vi "hw4-2 topVI.vi"() -> ()   [LabVIEW 2014]
uses:
  <vilib>/regexp/Match Regular Expression.xnode
panel:
  in  "file path (use dialog)":path
  out "output":string[][](array[string])
  in  "Firewall log raw data":string="Apr 26 21:31:34 filterlog: 129,16777216,,1425041642,hn0,match,pass,in,4,0x0,,128,16110,0,none,17,udp,36,10.2.10.175,255.255.255.255,60221,3956,16\nApr 26 21:31:34 filterlog: 129,16777216,,1425041642,hn0,match,pass,in,4,0x0,,128,4117,0,none,17,udp,78,10.2.10.1,208.93.4.206,137,137,58\nApr 26 21:31:32 filterlog: 130,16777216,,1425041643,hn0,match,pass,in,4,0x0,,128,18168,0,DF,17,udp,351,10.2.10.10,10.2.23.123,53,59118,331\nApr 26 21:31:32 filterlog: 129,16777216,,1425041642,hn0,match,pass,in,4,0x0,,128,10627,0,none,17,udp,82,10.2.10.10,140.112.2.2,59087,53,62\nApr 26 21:31:32 filterlog: 129,16777216,,1425041642,hn0,match,pass,in,4,0x0,,128,10626,0,none,17,udp,98,10.2.10.10,140.112.2.2,60847,53,78\nApr 26 21:38:10 filterlog: 105,16777216,,1425041627,hn1,match,block,in,4,0x2,0,109,9812,0,DF,6,tcp,48,207.46.13.171,10.2.10.15,25309,80,0,SEC,27892632,,8192,,mss;nop;nop;sackOK\nApr 26 21:38:08 filterlog: 129,16777216,,1425041642,hn0,match,pass,in,4,0x0,,128,23124,0,DF,6,tcp,52,10.2.10.172,207.46.153.155,60590,443,0,S,2141064781,,8192,,mss;nop;wscale;nop;nop;sackOK\nApr 26 21:38:08 filterlog: 130,16777216,,1425041643,hn0,match,block,in,4,0x2,0,128,8596,0,DF,6,tcp,48,10.2.10.2,10.2.102.10,41875,88,0,SEC,3256166066,,8192,,mss;nop;nop;sackOK\nApr 26 21:38:07 filterlog: 130,16777216,,1425041643,hn0,match,pass,in,4,0x2,0,128,8592,0,DF,6,tcp,48,10.2.10.2,10.2.102.10,41874,88,0,SEC,2184502132,,8192,,mss;nop;nop;sackOK"
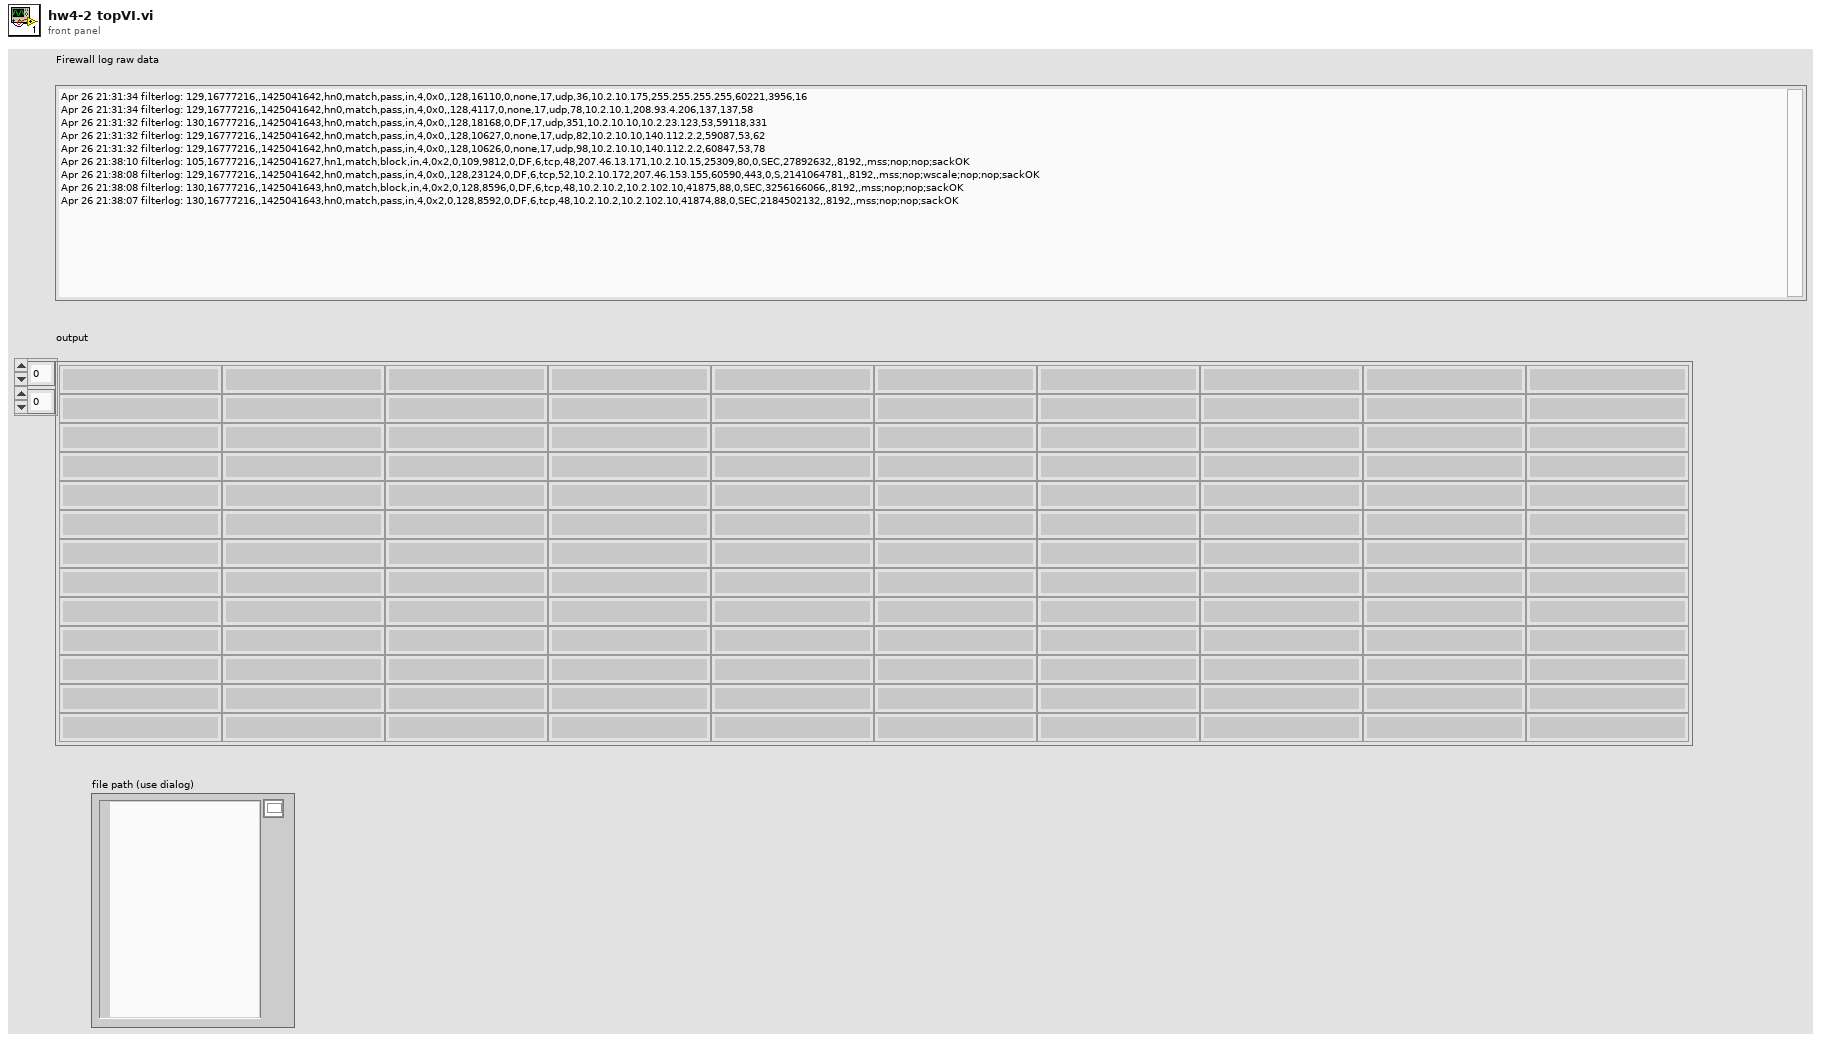
[diagram p1: front panel]
types:
  T1 = enum16{"open", "replace", "create", "open or create", "replace or create", "replace or create with confirmation"}
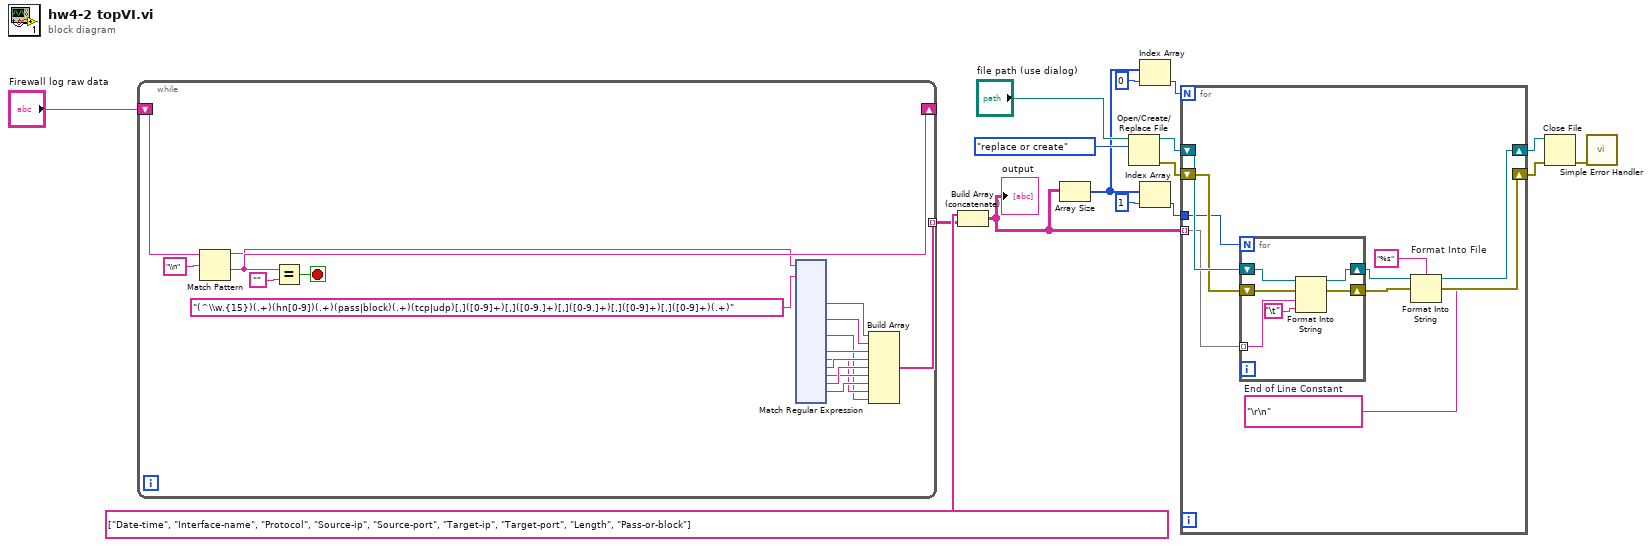
[diagram p0: block diagram]
diagram:
  n1 = while {
    shift-right: [w31] -> _
    shift-left: "Firewall log raw data" -> [w33]
    tunnel: [w17] -> w14 mode=indexing
    stop <- w29 stop-if-true
    n2 = Match Pattern(string=w33, regular expression="\\n") -> (before substring=w28:string, after substring=w31:string)  [unwired: 1 in, 2 out]
    n3 = Equal?(x=w31, y="") -> (x = y?=w29:bool)
    n4 = xnode "Match Regular Expression"("input string"=w28, "regular expression"="(^\\w.{15})(.+)(hn[0-9])(.+)(pass|block)(.+)(tcp|udp)[,]([0-9]+)[,]([0-9.]+)[,]([0-9.]+)[,]([0-9]+)[,]([0-9]+)(.+)") -> ("submatch 1"=w26:string, "submatch 3"=w25:string, "submatch 5"=w18:string, "submatch 7"=w24:string, "submatch 8"=w19:string, "submatch 9"=w23:string, "submatch 10"=w21:string, "submatch 11"=w22:string, "submatch 12"=w20:string)  [unwired: 4 in, 9 out]
    n5 = Build Array(w26, w25, w24, w23, w22, w21, w20, w19, w18) -> (w17:string[])
  }
  n6 = Build Array (concatenate)(string[] ["Date-time", "Interface-name", "Protocol", "Source-ip", "Source-port", "Target-ip", "Target-port", "Length", "Pass-or-block"], w14) -> (w1:string[][])
  "output" <- w1
  n7 = Array Size(array=w1) -> (size(s)=w5:i32[])
  n8 = Open/Create/Replace File(file path (use dialog)="file path (use dialog)", operation (0:open)=T1."replace or create") -> (refnum out=w11:refnum<file>, error out=w10:errorcluster)  [unwired: 4 in, 1 out]
  n9 = Index Array(array=w5, index=0) -> (element=w3:i32)
  n10 = Index Array(array=w5, index=1) -> (element=w2:i32)
  n11 = for {
    N: w3 -> [_]
    shift-right: [w166] -> w9
    shift-left: w11 -> [w171]
    shift-right: [w167] -> w8
    shift-left: w10 -> [w170]
    tunnel: w2 -> [w163]
    tunnel: w1 -> [w162] mode=indexing
    w164 = "\r\n"  # End of Line Constant
    n12 = for {
      N: w163 -> [_]
      shift-right: [w176] -> w169
      shift-left: w171 -> [w177]
      shift-right: [w174] -> w168
      shift-left: w170 -> [w175]
      tunnel: w162 -> [w173] mode=indexing
      n13 = Format Into String(initial string=w177, error in=w175, w173, "\t") -> (resulting string=w176:refnum<file>, error out=w174:errorcluster)  [unwired: 1 in]
    }
    n14 = Format Into String "Format Into File"(format string="%s", initial string=w169, error in=w168, w164) -> (resulting string=w166:refnum<file>, error out=w167:errorcluster)
  }
  n15 = Close File(refnum=w9, error in=w8) -> (error out=w7:errorcluster)  [unwired: 1 out]
  n16 = call <vilib>:"Simple Error Handler.vi"("error in (no error)"=w7) -> ()  [unwired: 4 in, 5 out]
